vi "Callback Template.vi"(8 "error in (no error)":errorcluster, 9 "Scope":variant, 11 "Value in":variant) -> (0 "error out":errorcluster)   [LabVIEW 2017]
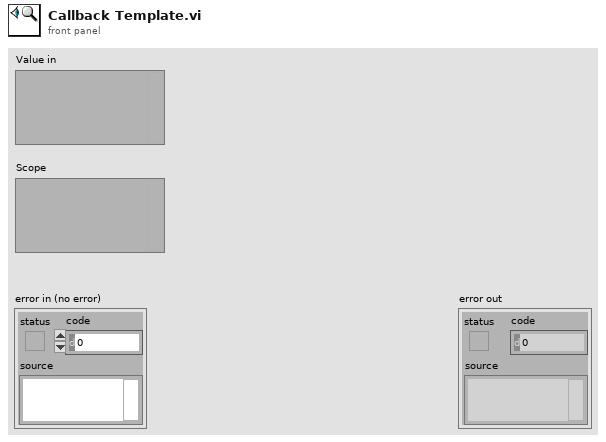
[diagram p1: front panel]
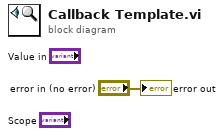
[diagram p0: block diagram]
diagram:
  "error out" <- "error in (no error)"
